vi "Add Data Section.vi"(8 "error in (no error)":errorcluster, 11 "Item Ref in":T1 format="%.0x") -> (0 "error out":errorcluster, 2 "Data Section Ptr":T1 format="%.0x", 3 "Item Ref out":T1 format="%.0x")   [LabVIEW 2017, in "DSF System Explorer.lvlib"]
uses:
  DSF System Explorer.lvlib
  <vilib>/NI Veristand/Custom Device API/Custom Device Item Ref.ctl
  Shared/Data Section Page GUID.vi
  <vilib>/NI Veristand/Custom Device API/Custom Device API.lvlib
  Shared/DSF Shared.lvlib
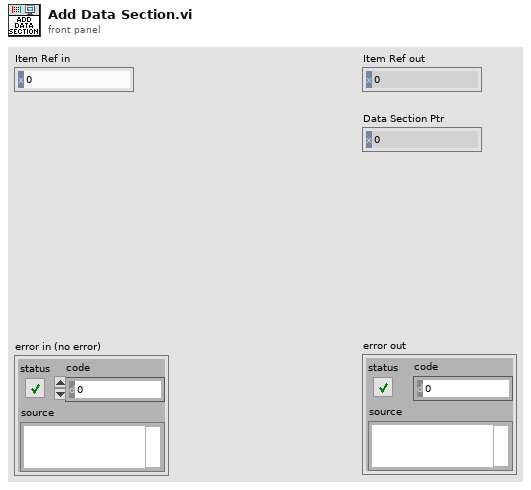
[diagram p1: front panel]
types:
  T1 = typedef "Custom Device API.lvlib/Custom Device Item Ref.ctl" = u64
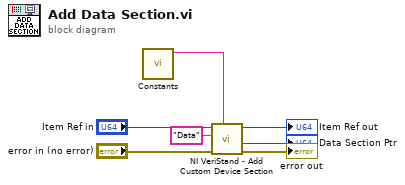
[diagram p0: block diagram]
diagram:
  n1 = call-poly "Constants.vi"() -> ("Data GUID"=w2:string)  [unwired: 11 in]
  n2 = call <vilib>:"NI VeriStand - Add Custom Device Section.vi"("GUID (Default Section)"=w2, "error in (no error)"="error in (no error)", "Section Name"="Data", "Parent Ref in"="Item Ref in") -> ("error out"=→"error out":errorcluster, "Section Ptr"=→"Data Section Ptr":T1, "Parent Ref out"=→"Item Ref out":T1)  [unwired: 4 in, 1 out]
